vi "Symbol Map.vi"() -> (3 "symbol_map":cdb[](array[numeric]))   [LabVIEW 2013]
uses:
  <vilib>/imath/engines/lvmath2/RunTimeEngine/NodeEndStatement/NIMS_NodeEndStatement_Output.vi
  <instcachedir>/0/NIMS_NodeEndStatement_Output_53EC0D466D134D7ABD903AC30B43404B.lvgen/NIMS_NodeEndStatement_Output_53EC0D466D134D7ABD903AC30B43404B_000.vi
  <vilib>/imath/engines/lvmath2/RunTimeEngine/ErrorHandling/NIMS_Finalize Error.vi
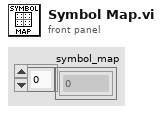
[diagram p1: front panel]
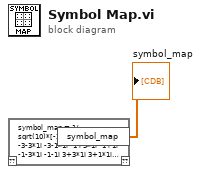
[diagram p0: block diagram]
diagram:
  n1 = mathscript code="symbol_map = 1/sqrt(10)*[-3+3*1i -3+1*1i -3-3*1i -3-1*1i -1+3*1i -1+1i -1-3*1i -1-1i 3+3*1i 3+1*1i 3-3*1i 3-1*1i 1+3*1i 1+1*1i 1-3*1i 1-1*1i];"() -> ("symbol_map"=→"symbol_map":cdb[])  [unwired: 1 in, 1 out]
